vi "Move translation stage.vi"() -> ()   [LabVIEW 2013]
uses:
  <vilib>/Utility/file.llb/Read From Spreadsheet File (I64).vi
  <vilib>/Utility/file.llb/Write To Spreadsheet File (DBL).vi
  Drivers and libraries/Zaber A Series/Zaber A Series.lvlib
panel:
  in  "Speed (fast mode only)":string="76800"
  in  "Fast":bool
  in  "Device number":string="01"
  in  "Load saved position":bool=TRUE
  in  "Save position":bool=TRUE
  in  "Path for saved position":path=path "C:/Users/lab/Documents/GitHub/single-photon-vision/LabVIEW 2013 SP1/Tools/Calibration/position-translation.txt"
  in  "Step Size":i32=1000
  out "error out":errorcluster
  in  "error in (no error)":errorcluster
  in  "VISA resource name":refnum<visa-resource-name>="COM5"
  in  "stop":bool
  out "Current position":dbl
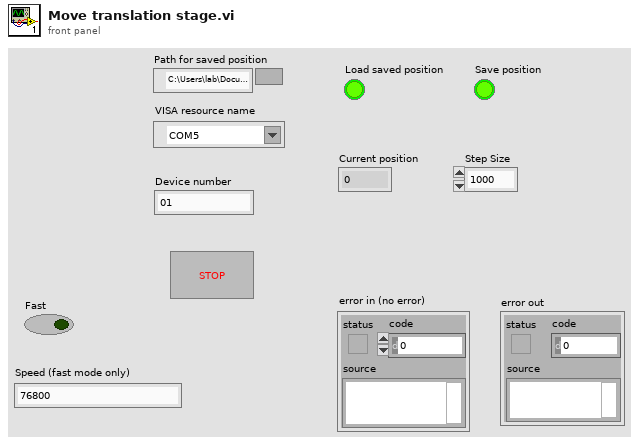
[diagram p1: front panel]
types:
  T1 = enum16{"0", "1", "2", "3", "4", "5", "6", "7", "8", "9", "A", "B", "C", "D", "E", "F", "G", "H", "I", "J", "K", "L", "M", "N", "O", "P", "Q", "R", "S", "T", "U", "V", "W", "X", "Y", "Z", "F1", "F2", "F3", "F4", "F5", "F6", "F7", "F8", "F9", "F10", "F11", "F12", "F13", "F14", "F15", "ADD", "BACK", "BACKSLASH", "CAPITAL", "COMMA", "DECIMAL", "DELETE", "DIVIDE", "DOWN", "END", "EQUALS", "ESCAPE", "GRAVE (`)", "HOME", "INSERT", "LBRACKET", "LCONTROL", "LEFT", "L ALT", "LSHIFT", "LWIN", "MINUS", "MULTIPLY", "NEXT", "NUMLOCK", "NUMPAD_0", "NUMPAD_1", "NUMPAD_2", "NUMPAD_3", "NUMPAD_4", "NUMPAD_5", "NUMPAD_6", "NUMPAD_7", "NUMPAD_8", "NUMPAD_9", "PAUSE", "PERIOD", "PRIOR (PG UP)", "RBRACKET", "RCONTROL", "RETURN", "RIGHT", "R ALT", "RSHIFT", "RWIN", "SCROLL", "SEMICOLON", "SLASH", "SPACE", "SUBTRACT", "TAB", "UP", "ENTER (num pad)", "' (quote)"}
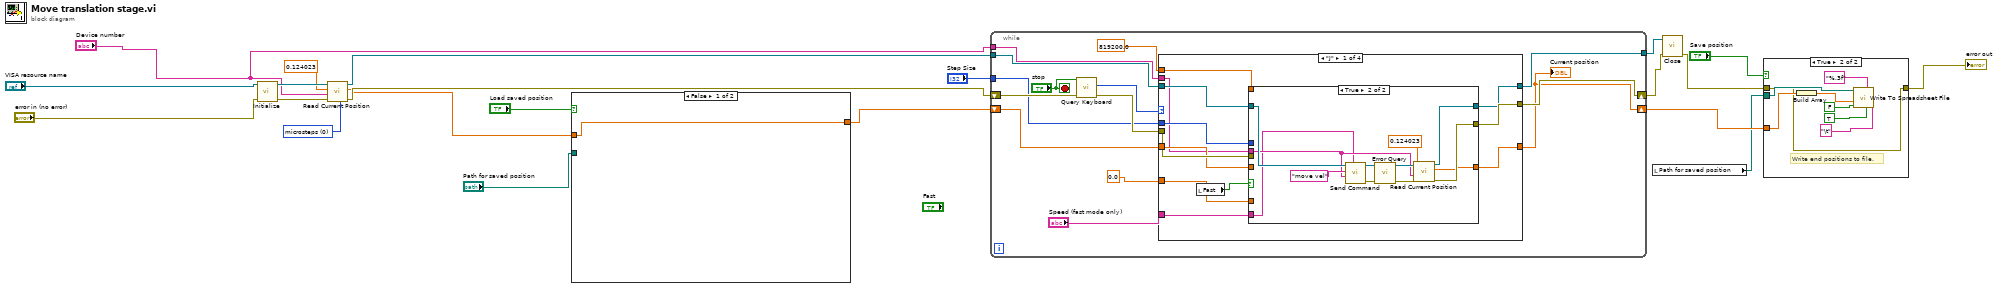
[diagram p0: block diagram]
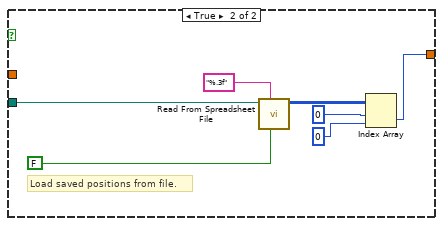
[diagram p3: hidden frame]
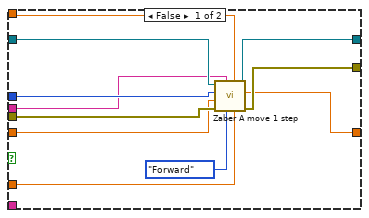
[diagram p4: hidden frame]
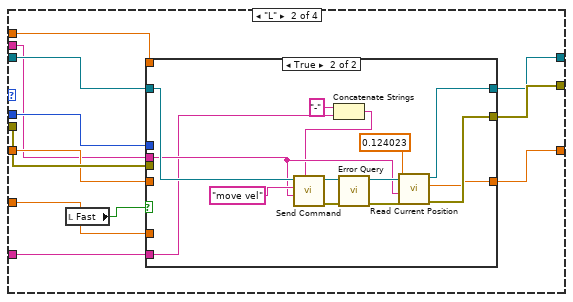
[diagram p5: hidden frame]
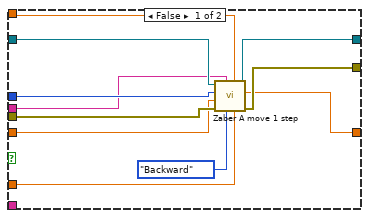
[diagram p6: hidden frame]
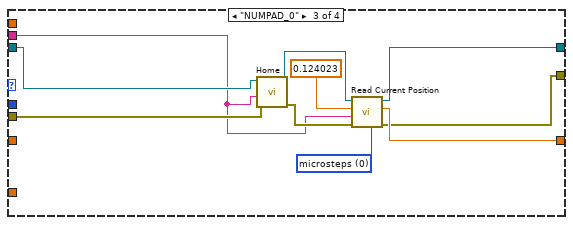
[diagram p7: hidden frame]
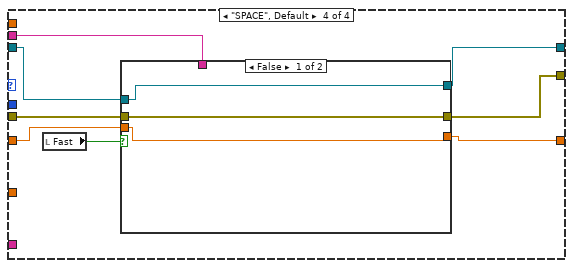
[diagram p8: hidden frame]
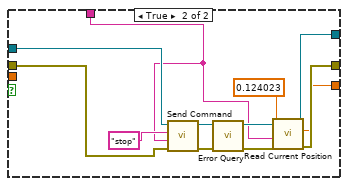
[diagram p9: hidden frame]
diagram:
  w4 = u16 0 items=["microsteps", "microns", "millimeters", "inches"] ("Units (0: microsteps)")
  n1 = call "Initialize.vi"("error in (no error)"="error in (no error)", "VISA resource name"="VISA resource name") -> ("error out"=w8:errorcluster, "VISA resource name out"=w6:refnum<visa-resource-name>)  [unwired: 8 in]
  n2 = call "Read Current Position.vi"("Units (0: microsteps)"=w4, "error in (no error)"=w8, "Device and Axis"="Device number", "Microstep Size (0)"=0.124023, "VISA resource name"=w6) -> ("error out"=w7:errorcluster, "Position"=w2:dbl, "VISA resource name out"=w3:refnum<visa-resource-name>)  [unwired: 4 in]
  n3 = case shown="False" "Load saved position" {
    tunnel: "Path for saved position" -> [_ w29]
    tunnel: [w22 w24] -> w15
    tunnel: w2 -> [w22 _]
    frame False {
    }
    frame True {
      # "Load saved positions from file."
      n4 = call-poly <vilib>:"Read From Spreadsheet File.vi"("transpose (no:F)"=FALSE, "format (%d)"="%.3f" ("format (%.3f)"), "file path (dialog if empty)"=w29) -> ("all rows"=w23:i64[][])  [unwired: 4 in, 4 out]
      n5 = Index Array(array=w23, index (row)=0 ("index"), index (col)=0 ("disabled index (col)")) -> (element=w24:i64)
    }
  }
  n6 = while {
    shift-right: [w41] -> w12
    shift-left: w7 -> [w43]
    tunnel: "Step Size" -> [w39]
    tunnel: "Device number" -> [w38]
    tunnel: w3 -> [w37]
    tunnel: [w36] -> w10
    shift-right: [w33] -> w20
    shift-left: w15 -> [w34]
    stop <- "stop" stop-if-true
    n7 = call "Query Keyboard.vi"("error in (no error)"=w43, "Stop?"="stop") -> ("error out"=w42:errorcluster, "element"=w40:T1)  [unwired: 8 in]
    n8 = case shown="\"J\"" w40 {
      tunnel: w42 -> [w55 w90 w124 w130]
      tunnel: [w54 w89 w116 w129] -> w41
      tunnel: w37 -> [w53 w88 w125 w128]
      tunnel: w39 -> [w52 w87 _ _]
      tunnel: w38 -> [w50 w85 w120 w126]
      tunnel: [w48 w83 w118 w127] -> w36
      tunnel: 819200.0 ("Data") -> [w49 w84 _ _]
      tunnel: w34 -> [w51 w86 _ w132]
      tunnel: [w47 w82 w117 w131] -> w33
      tunnel: 0.0 ("Minimum") -> [w46 w81 _ _]
      tunnel: "Speed (fast mode only)" -> [w44 w79 _ _]
      frame "J" {
        n9 = local read "Fast"() -> (w45:bool)
        n10 = case shown="True" w45 {
          tunnel: w55 -> [w66 _]
          tunnel: [w65 w69] -> w54
          tunnel: w53 -> [w64 w76]
          tunnel: w52 -> [w63 _]
          tunnel: w51 -> [w62 _]
          tunnel: w50 -> [w61 w72]
          tunnel: w49 -> [w60 _]
          tunnel: [w59 w70] -> w48
          tunnel: [w58 w68] -> w47
          tunnel: w46 -> [w56 _]
          tunnel: w44 -> [_ w67]
          frame False {
            n11 = call "Zaber A move 1 step.vi"("Minimum"=w56, "Maximum"=w60, "Direction"=enum16{"Forward", "Backward"}."Forward", "Device and Axis"=w61, "error in (no error)"=w66, "Current position in"=w62, "Step Size"=w63, "VISA Refnum in"=w64) -> ("error out"=w65:errorcluster, "Position"=w58:dbl, "VISA Refnum out"=w59:refnum<visa-resource-name>)  [unwired: 1 in]
          }
          frame True {
            n12 = call "Send Command.vi"("Data"=w67, "Device and Axis"=w72, "Command"="move vel", "VISA resource name"=w76) -> ("error out"=w77:errorcluster, "VISA resource name out"=w78:refnum<visa-resource-name>)  [unwired: 3 in, 3 out]
            n13 = call "Error Query.vi"("error in (no error)"=w77, "VISA resource name"=w78) -> ("error out"=w73:errorcluster, "VISA resource name out"=w74:refnum<visa-resource-name>)  [unwired: 6 in, 2 out]
            n14 = call "Read Current Position.vi"("error in (no error)"=w73, "Device and Axis"=w72, "Microstep Size (0)"=0.124023, "VISA resource name"=w74) -> ("error out"=w69:errorcluster, "Position"=w68:dbl, "VISA resource name out"=w70:refnum<visa-resource-name>)  [unwired: 5 in]
          }
        }
      }
      frame "L" {
        n15 = local read "Fast"() -> (w80:bool)
        n16 = case shown="True" w80 {
          tunnel: w90 -> [w101 _]
          tunnel: [w100 w106] -> w89
          tunnel: w88 -> [w99 w113]
          tunnel: w87 -> [w98 _]
          tunnel: w86 -> [w97 _]
          tunnel: w85 -> [w96 w109]
          tunnel: w84 -> [w95 _]
          tunnel: [w94 w107] -> w83
          tunnel: [w93 w105] -> w82
          tunnel: w81 -> [w91 _]
          tunnel: w79 -> [_ w104]
          frame False {
            n17 = call "Zaber A move 1 step.vi"("Minimum"=w91, "Maximum"=w95, "Direction"=enum16{"Forward", "Backward"}."Backward", "Device and Axis"=w96, "error in (no error)"=w101, "Current position in"=w97, "Step Size"=w98, "VISA Refnum in"=w99) -> ("error out"=w100:errorcluster, "Position"=w93:dbl, "VISA Refnum out"=w94:refnum<visa-resource-name>)  [unwired: 1 in]
          }
          frame True {
            n18 = Concatenate Strings("-" ("string"), w104) -> (w102:string)
            n19 = call "Send Command.vi"("Data"=w102, "Device and Axis"=w109, "Command"="move vel", "VISA resource name"=w113) -> ("error out"=w114:errorcluster, "VISA resource name out"=w115:refnum<visa-resource-name>)  [unwired: 3 in, 3 out]
            n20 = call "Error Query.vi"("error in (no error)"=w114, "VISA resource name"=w115) -> ("error out"=w110:errorcluster, "VISA resource name out"=w111:refnum<visa-resource-name>)  [unwired: 6 in, 2 out]
            n21 = call "Read Current Position.vi"("error in (no error)"=w110, "Device and Axis"=w109, "Microstep Size (0)"=0.124023, "VISA resource name"=w111) -> ("error out"=w106:errorcluster, "Position"=w105:dbl, "VISA resource name out"=w107:refnum<visa-resource-name>)  [unwired: 5 in]
          }
        }
      }
      frame "NUMPAD_0" {
        w119 = u16 0 items=["microsteps", "microns", "millimeters", "inches"] ("Units (0: microsteps)")
        n22 = call "Home.vi"("error in (no error)"=w124, "Device and Axis"=w120, "VISA resource name"=w125) -> ("error out"=w122:errorcluster, "VISA resource name out"=w123:refnum<visa-resource-name>)  [unwired: 7 in]
        n23 = call "Read Current Position.vi"("Units (0: microsteps)"=w119, "error in (no error)"=w122, "Device and Axis"=w120, "Microstep Size (0)"=0.124023, "VISA resource name"=w123) -> ("error out"=w116:errorcluster, "Position"=w117:dbl, "VISA resource name out"=w118:refnum<visa-resource-name>)  [unwired: 4 in]
      }
      frame "SPACE", Default {
        n24 = local read "Fast"() -> (w133:bool)
        n25 = case shown="False" w133 {
          tunnel: [w136 w141] -> w131
          tunnel: w132 -> [w136 _]
          tunnel: w130 -> [w135 w137]
          tunnel: [w135 w142] -> w129
          tunnel: w128 -> [w134 w140]
          tunnel: [w134 w139] -> w127
          tunnel: w126 -> [_ w138]
          frame False {
          }
          frame True {
            n26 = call "Send Command.vi"("error in (no error)"=w137, "Device and Axis"=w138, "Command"="stop", "VISA resource name"=w140) -> ("error out"=w147:errorcluster, "VISA resource name out"=w148:refnum<visa-resource-name>)  [unwired: 3 in, 3 out]
            n27 = call "Error Query.vi"("error in (no error)"=w147, "VISA resource name"=w148) -> ("error out"=w144:errorcluster, "VISA resource name out"=w145:refnum<visa-resource-name>)  [unwired: 6 in, 2 out]
            n28 = call "Read Current Position.vi"("error in (no error)"=w144, "Device and Axis"=w138, "Microstep Size (0)"=0.124023, "VISA resource name"=w145) -> ("error out"=w142:errorcluster, "Position"=w141:dbl, "VISA resource name out"=w139:refnum<visa-resource-name>)  [unwired: 5 in]
          }
        }
      }
    }
    "Current position" <- w33
  }
  n29 = local read "Path for saved position"() -> (w9:path)
  n30 = call "Close.vi"("error in (no error)"=w12, "VISA resource name"=w10) -> ("error out"=w11:errorcluster)  [unwired: 9 in]
  n31 = case shown="True" "Save position" {
    tunnel: w20 -> [_ w157]
    tunnel: w9 -> [_ w156]
    tunnel: w11 -> [w149 w150]
    tunnel: [w149 w150] -> w19
    frame False {
    }
    frame True {
      # "Write end positions to file."
      n32 = Build Array(w157) -> (w151:dbl[])
      n33 = call-poly <vilib>:"Write To Spreadsheet File.vi"("delimiter (\\t)"="\t" ("delimiter (\\t)"), "transpose? (no:F)"=TRUE, "format (%.3f)"="%.3f", "append to file? (new file:F)"=FALSE, "1D data"=w151, "file path (dialog if empty)"=w156) -> ()  [unwired: 2 in, 1 out]
    }
  }
  "error out" <- w19
